vi "Start Module Interface.vi"(8 "error in (no error)":errorcluster, 10 "rSubPanel":refnum<vi>, 11 "模块定义":T1={"模块名称"="系统", "项定义"=[{"项名"="设置", "符号图形路径"=path "D:/GitHub/UI-Frame/Pictures/Setting.png"}, {"项名"="帮助", "符号图形路径"=path "D:/GitHub/UI-Frame/Pictures/Help.png"}]}) -> (0 "error out":errorcluster, 3 "模块名称":string)   [LabVIEW 2020, in "Grouped Interface.lvlib"]
uses:
  Grouped Interface.lvlib
  Module Definition--cluster.ctl
  Function Item--cluster.ctl
  Module Interface.vi
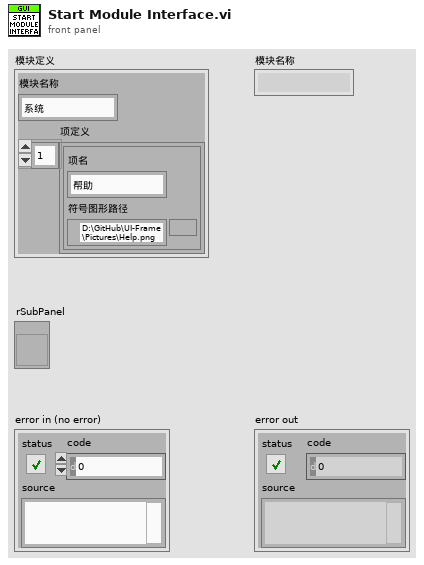
[diagram p1: front panel]
types:
  T1 = typedef "Grouped Interface.lvlib/Module Definition--cluster.ctl" = cluster{"模块名称":string, "项定义":T2[]}
  T2 = typedef "Grouped Interface.lvlib/Function Item--cluster.ctl" = cluster{"项名":string, "符号图形路径":path}
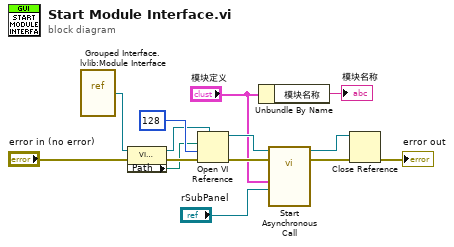
[diagram p0: block diagram]
diagram:
  n1 = vi-ref "Grouped Interface.lvlib:Module Interface.vi"() -> (w7:refnum<vi>)
  n2 = property class="VI (strict)"(reference=w7, error in="error in (no error)") -> (reference out=w11:refnum<vi>, error out=w9:errorcluster, "Path"=w8:path)
  n3 = Open VI Reference(type specifier VI Refnum (for type only)=w11, vi path=w8, options=128, error in (no error)=w9) -> (vi reference=w10:refnum<vi>, error out=w6:errorcluster)  [unwired: 2 in]
  n4 = Unbundle By Name("模块定义") -> ("模块名称"=→"模块名称":string)
  n5 = call-by-ref "Start Asynchronous Call"(reference=w10, error in=w6, "rSubPanel"="rSubPanel", "模块定义"="模块定义") -> (reference out=w13:refnum<vi>, error out=w12:errorcluster)  [unwired: 10 in]
  n6 = Close Reference(reference=w13, error in (no error)=w12) -> (error out=→"error out":errorcluster)
